vi "FadeLeftRight.vi"(11 "Key":string) -> ()   [LabVIEW 2022 SP3]
uses:
  Mic/Mic_Global.vi
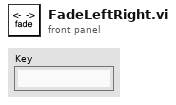
[diagram p1: front panel]
types:
  T1 = cluster{"Alerts":bool, "Log X Axis":bool, "dB scale":bool, "Averaging":bool, "Fade":dbl, "Centroids?":bool}
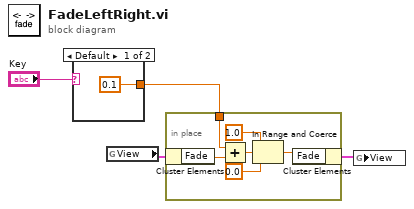
[diagram p0: block diagram]
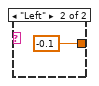
[diagram p2: hidden frame]
diagram:
  n1 = case shown="Default" "Key" {
    tunnel: [0.1 -0.1] -> w4
    frame Default {
    }
    frame "Left" {
    }
  }
  n2 = global read "Mic_Global.vi" "View"() -> (w2:T1)
  n3 = in-place {
    in-place-border: w4 -> [w11]
    n4 = in-place-cluster #1(w2) -> ("Fade"=w12:dbl)
    n5 = Add(x=w11, y=w12) -> (x+y=w10:dbl)
    n6 = In Range and Coerce(upper limit=1.0, x=w10, lower limit=0.0) -> (coerced(x)=w9:dbl)  [unwired: 1 out]
    n7 = in-place-cluster #1("Fade"=w9) -> (w1:T1)
  }
  n8 = global write "Mic_Global.vi" "View"(w1) -> ()
